vi "add glyphs.vi"(8 "error in":errorcluster, 9 "glyphs":T1[](array[typedef]), 10 "names":string[](array[string]), 11 "glyph manager in":T2) -> (0 "error out":errorcluster, 3 "glyph manager out":T2)   [LabVIEW 2025, in "CEF.lvlib"]
doc: "Copyright 2017 National Instruments Corporation\n\nLicensed under the Apache License, Version 2.0 (the \"License\"); you may not use this file except in compliance with the License. You may obtain a copy of the License at http://www.apache.org/licenses/LICENSE-2.0\nUnless required by applicable law or agreed to in writing, software distributed under the License is distributed on an \"AS IS\" BASIS, WITHOUT WARRANTIES OR CONDITIONS OF ANY KIND, either express or implied. See the License for the specific language governing permissions and limitations under the License."
uses:
  CEF.lvlib
  glyph manager.ctl
  <vilib>/picture/picture.llb/imagedata.ctl
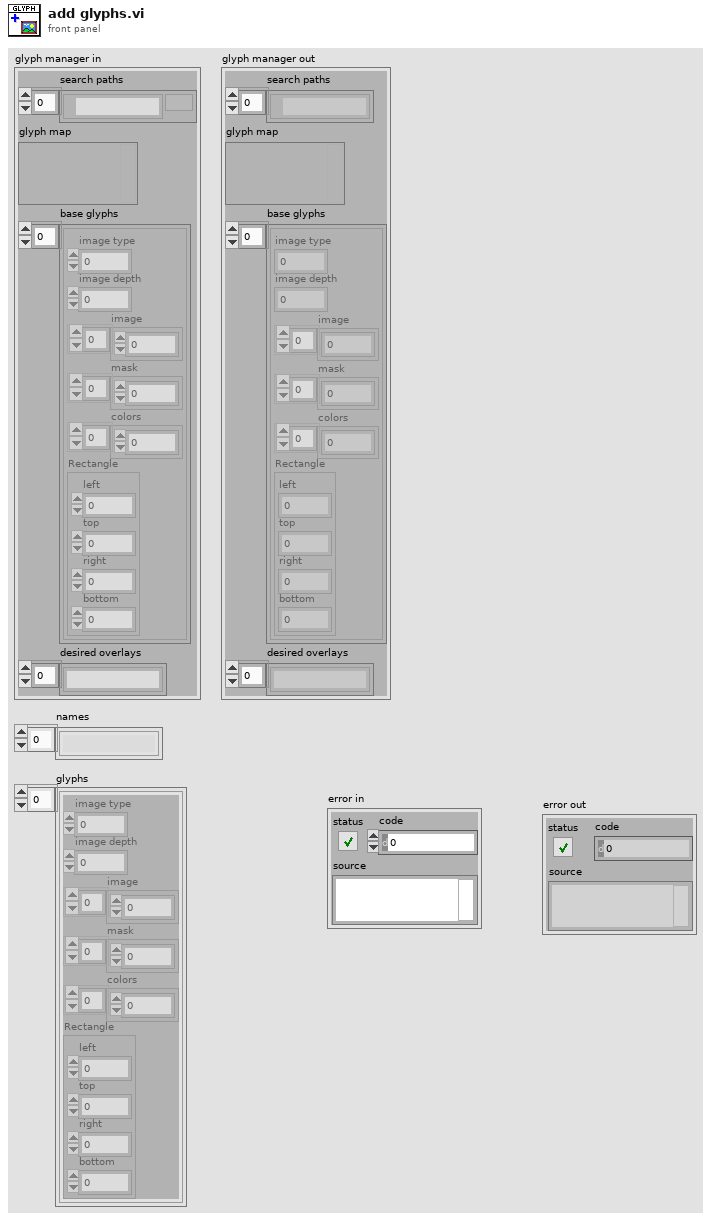
[diagram p1: front panel]
types:
  T1 = typedef "imagedata.ctl" = cluster{"image type":i32, "image depth":i32, "image":u8[], "mask":u8[], "colors":u32[], "Rectangle":cluster{"left":i16, "top":i16, "right":i16, "bottom":i16}}
  T2 = typedef "CEF.lvlib/glyph manager.ctl" = cluster{"search paths":path[], "glyph map":variant, "base glyphs":T1[], "desired overlays":string[]}
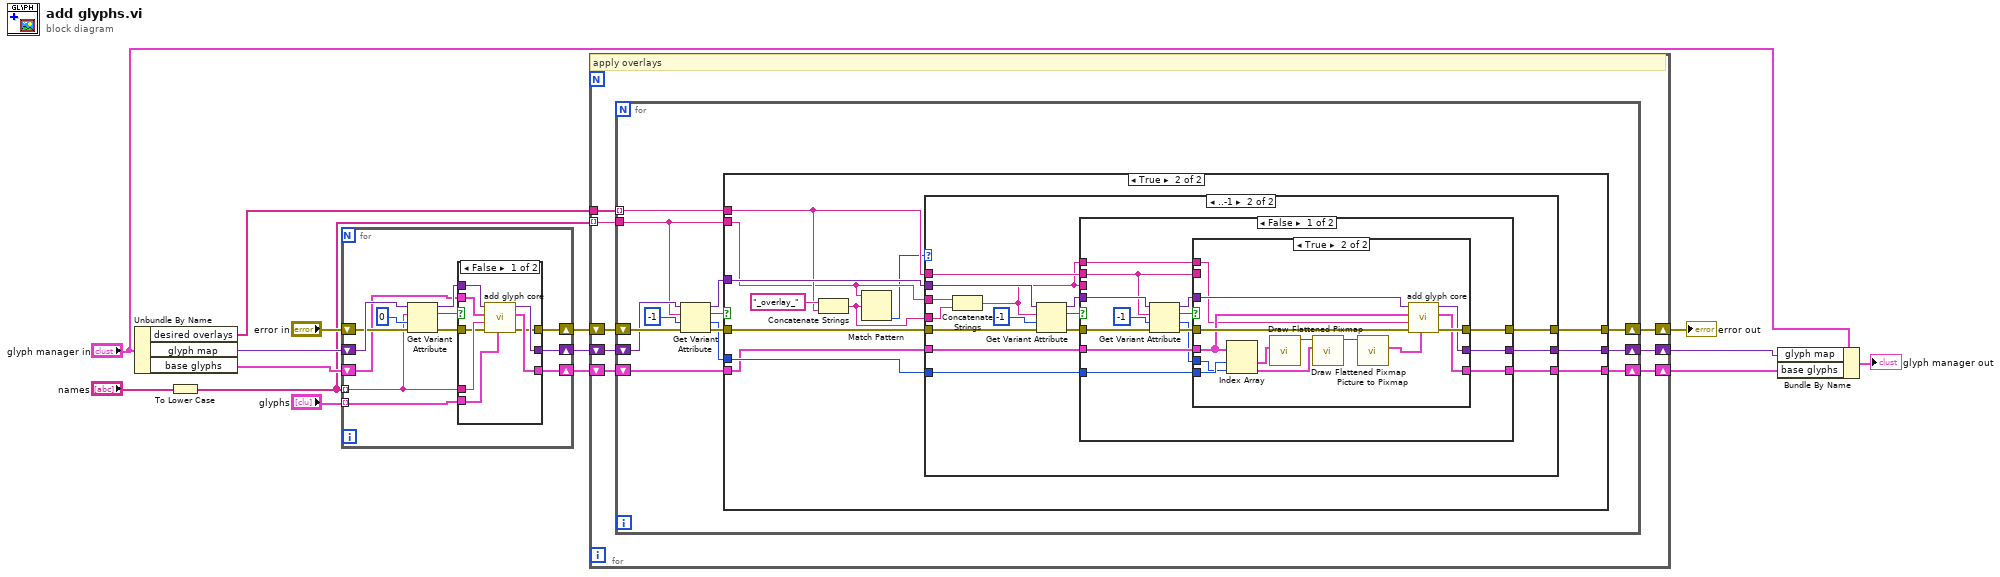
[diagram p0: block diagram]
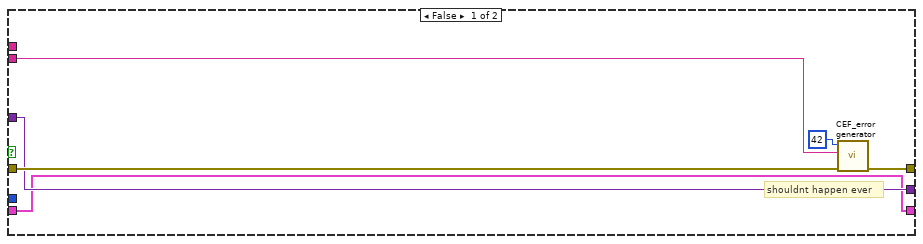
[diagram p2: hidden frame]
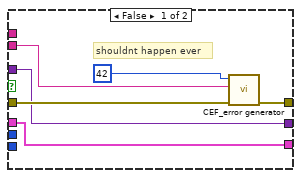
[diagram p4: hidden frame]
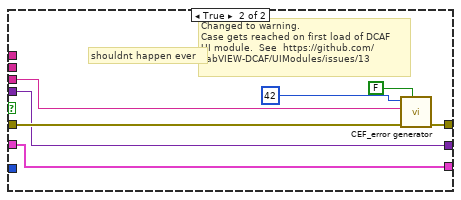
[diagram p5: hidden frame]
diagram:
  n1 = Unbundle By Name("glyph manager in") -> ("desired overlays"=w4:string[], "glyph map"=w13:variant, "base glyphs"=w14:T1[])
  n2 = To Lower Case(string="names") -> (all lower case string=w1:string[])
  n3 = for {
    shift-right: [w21] -> w8
    shift-left: w13 -> [w27]
    shift-right: [w18] -> w7
    shift-left: w14 -> [w19]
    shift-right: [w23] -> w9
    shift-left: "error in" -> [w25]
    tunnel: w1 -> [w16] mode=indexing
    tunnel: "glyphs" -> [w17] mode=indexing
    n4 = Get Variant Attribute(Variant=w27, name=w16, default value (empty Variant)=0, error in=w25) -> (duplicate Variant=w20:variant, found=w24:bool, error out=w22:errorcluster)  [unwired: 1 out]
    n5 = case shown="False" w24 {
      tunnel: [w29 w38] -> w23
      tunnel: w22 -> [w30 w38]
      tunnel: [w34 w37] -> w21
      tunnel: w20 -> [w31 w37]
      tunnel: w19 -> [w35 w36]
      tunnel: [w33 w36] -> w18
      tunnel: w16 -> [w32 _]
      tunnel: w17 -> [w28 _]
      frame False {
        n6 = call "add glyph core.vi"("image data"=w28, "error in"=w30, "name"=w32, "base glyphs"=w35, "map in"=w31) -> ("error out"=w29:errorcluster, "base glyphs out"=w33:T1[], "map out"=w34:variant)  [unwired: 4 in]
      }
      frame True {
      }
    }
  }
  n7 = for {
    shift-right: [w41] -> w6
    shift-left: w8 -> [w42]
    shift-right: [w39] -> w5
    shift-left: w7 -> [w40]
    tunnel: w4 -> [w46]
    tunnel: w1 -> [w45] mode=indexing
    shift-right: [w43] -> w2
    shift-left: w9 -> [w44]
    # "apply overlays"
    n8 = for {
      tunnel: w46 -> [w48] mode=indexing
      tunnel: w45 -> [w49]
      shift-right: [w54] -> w43
      shift-left: w44 -> [w59]
      shift-right: [w52] -> w41
      shift-left: w42 -> [w58]
      shift-right: [w50] -> w39
      shift-left: w40 -> [w51]
      n9 = Get Variant Attribute(Variant=w58, name=w49, default value (empty Variant)=-1, error in=w59) -> (duplicate Variant=w53:variant, found=w56:bool, value=w47:i32, error out=w55:errorcluster)
      n10 = case shown="True" w56 {
        tunnel: w55 -> [w65 w76]
        tunnel: [w64 w74] -> w54
        tunnel: w53 -> [w62 w77]
        tunnel: [w62 w73] -> w52
        tunnel: w51 -> [w61 w69]
        tunnel: [w61 w72] -> w50
        tunnel: w49 -> [w60 w68]
        tunnel: w48 -> [_ w70]
        tunnel: w47 -> [_ w71]
        frame False {
          # "shouldnt happen ever"
          n11 = call "CEF_error generator.vi"("error in"=w65, "append error message"=w60, "error code (0)"=42) -> ("error out"=w64:errorcluster)  [unwired: 6 in]
        }
        frame True {
          n12 = Concatenate Strings("_overlay_" ("string"), w70) -> (w67:string)
          n13 = Match Pattern(string=w68, regular expression=w67) -> (offset past match=w66:i32)  [unwired: 1 in, 3 out]
          n14 = case shown="..-1" w66 {
            tunnel: w77 -> [w79 w95]
            tunnel: w76 -> [w80 w94]
            tunnel: [w80 w90] -> w74
            tunnel: [w79 w89] -> w73
            tunnel: [w78 w87] -> w72
            tunnel: w71 -> [_ w86]
            tunnel: w70 -> [_ w85]
            tunnel: w69 -> [w78 w84]
            tunnel: w68 -> [_ w82]
            tunnel: w67 -> [_ w81]
            frame 0.. {
              # "ok, just means its already an overlay"
            }
            frame ..-1 {
              n15 = Concatenate Strings(w82, w81) -> (w83:string)
              n16 = Get Variant Attribute(Variant=w95, name=w83, default value (empty Variant)=-1, error in=w94) -> (duplicate Variant=w88:variant, found=w92:bool, error out=w91:errorcluster)  [unwired: 1 out]
              n17 = case shown="False" w92 {
                tunnel: w91 -> [w108 w135]
                tunnel: [w104 w134] -> w90
                tunnel: [w102 w133] -> w89
                tunnel: w88 -> [w109 w133]
                tunnel: w84 -> [w100 w132]
                tunnel: [w99 w132] -> w87
                tunnel: w86 -> [w97 _]
                tunnel: w85 -> [w103 _]
                tunnel: w83 -> [_ w131]
                tunnel: w83 -> [w96 _]
                frame False {
                  n18 = Get Variant Attribute(Variant=w109, name=w103, default value (empty Variant)=-1, error in=w108) -> (duplicate Variant=w101:variant, found=w106:bool, value=w98:i32, error out=w105:errorcluster)
                  n19 = case shown="True" w106 {
                    tunnel: w105 -> [w114 w122]
                    tunnel: [w113 w123] -> w104
                    tunnel: w103 -> [w112 _]
                    tunnel: [w111 w117] -> w102
                    tunnel: w101 -> [w111 w120]
                    tunnel: w100 -> [w110 w121]
                    tunnel: [w110 w116] -> w99
                    tunnel: w98 -> [_ w126]
                    tunnel: w97 -> [_ w127]
                    tunnel: w96 -> [_ w119]
                    frame False {
                      # "shouldnt happen ever"
                      n20 = call "CEF_error generator.vi"("error in"=w114, "append error message"=w112, "error code (0)"=42) -> ("error out"=w113:errorcluster)  [unwired: 6 in]
                    }
                    frame True {
                      n21 = Index Array(array=w121, index #1=w127, index #2=w126) -> (element #1=w125:T1, element #2=w124:T1)
                      n22 = call <vilib>:"Draw Flattened Pixmap.vi"("image data"=w125) -> ("new picture"=w128:picture)  [unwired: 8 in]
                      n23 = call <vilib>:"Draw Flattened Pixmap.vi"("image data"=w124, "picture"=w128) -> ("new picture"=w129:picture)  [unwired: 7 in]
                      n24 = call <vilib>:"Picture to Pixmap.vi"("picture"=w129) -> ("image data"=w118:T1)  [unwired: 9 in, 1 out]
                      n25 = call "add glyph core.vi"("image data"=w118, "error in"=w122, "name"=w119, "base glyphs"=w121, "map in"=w120) -> ("error out"=w123:errorcluster, "base glyphs out"=w116:T1[], "map out"=w117:variant)  [unwired: 4 in]
                    }
                  }
                }
                frame True {
                  # "Changed to warning.\nCase gets reached on first load of DCAF\nUI module.  See  https://github.com/LabVIEW-DCAF/UIModules/issues/13"
                  # "shouldnt happen ever"
                  n26 = call "CEF_error generator.vi"("error (T)"=FALSE, "error in"=w135, "append error message"=w131, "error code (0)"=42) -> ("error out"=w134:errorcluster)  [unwired: 5 in]
                }
              }
            }
          }
        }
      }
    }
  }
  "error out" <- w2
  n27 = Bundle By Name(cluster="glyph manager in", "glyph map"=w6, "base glyphs"=w5) -> (→"glyph manager out":T2)
